vi "NF LI56xx sub get sig.vi"(7 "Type":string, 8 "error in":errorcluster caption="error in (no error)" {"code" format="%.0x"}, 10 "signal cluster":T1, 11 "VISA resource name":refnum<visa-resource-name>) -> (0 "error out":errorcluster {"code" format="%.0x"}, 2 "output":T1, 3 "VISA resource name copy":refnum<visa-resource-name>)   [LabVIEW 2019]
doc: "get input signal related parameters"
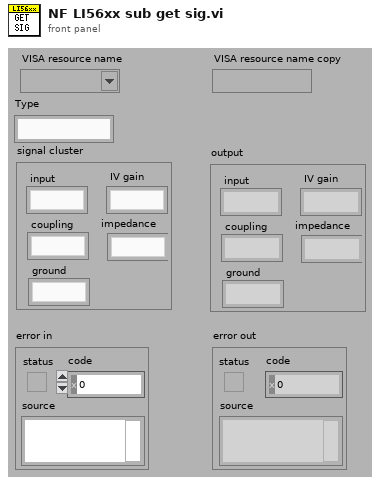
[diagram p1: front panel]
types:
  T1 = cluster{"input":string, "coupling":string, "ground":string, "IV gain":string, "impedance":string}
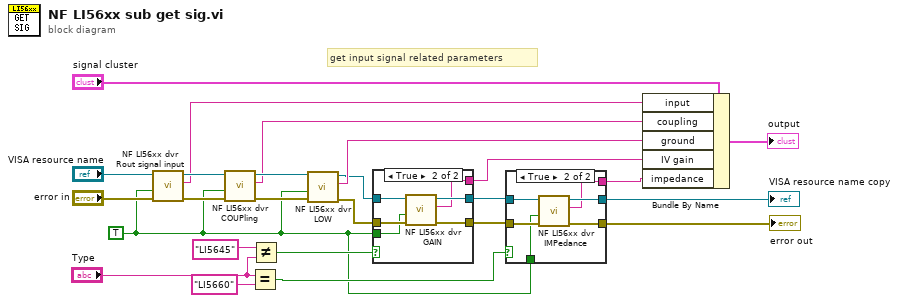
[diagram p0: block diagram]
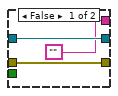
[diagram p2: hidden frame]
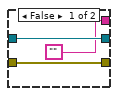
[diagram p3: hidden frame]
diagram:
  w1 = TRUE ("Read(F)")
  # "get input signal related parameters"
  n1 = call "NF LI56xx dvr Rout signal input.vi"("error in"="error in", "Read(F)"=w1, "VISA resource name"="VISA resource name") -> ("error out"=w23:errorcluster, "query signal input"=w19:string, "VISA resource name copy"=w25:refnum<visa-resource-name>)  [unwired: 6 in]
  n2 = call "NF LI56xx dvr COUPling.vi"("error in"=w23, "Read(F)"=w1, "VISA resource name"=w25) -> ("error out"=w22:errorcluster, "query coupling"=w18:string, "VISA resource name copy"=w24:refnum<visa-resource-name>)  [unwired: 6 in]
  n3 = Equal?(x="Type", y="LI5660") -> (x = y?=w8:bool)
  n4 = Not Equal?(x="LI5645" ("y"), y="Type") -> (x != y?=w7:bool)
  n5 = call "NF LI56xx dvr LOW.vi"("error in"=w22, "Read(F)"=w1, "VISA resource name"=w24) -> ("error out"=w4:errorcluster, "query grounding"=w17:string, "VISA resource name copy"=w5:refnum<visa-resource-name>)  [unwired: 6 in]
  n6 = case shown="True" w7 {
    tunnel: w5 -> [w28 w34]
    tunnel: w4 -> [w27 w33]
    tunnel: [w27 w32] -> w2
    tunnel: [w28 w31] -> w3
    tunnel: ["" w30] -> w6
    tunnel: w1 -> [_ w29]
    frame False {
    }
    frame True {
      n7 = call "NF LI56xx dvr GAIN.vi"("error in"=w33, "Read(F)"=w29, "VISA resource name"=w34) -> ("error out"=w32:errorcluster, "query IV gain"=w30:string, "VISA resource name copy"=w31:refnum<visa-resource-name>)  [unwired: 6 in]
    }
  }
  n8 = case shown="True" w8 {
    tunnel: w3 -> [w37 w43]
    tunnel: w2 -> [w36 w42]
    tunnel: [w36 w41] -> w13
    tunnel: [w37 w40] -> w12
    tunnel: ["" w39] -> w11
    tunnel: w1 -> [_ w38]
    frame False {
    }
    frame True {
      n9 = call "NF LI56xx dvr IMPedance.vi"("error in"=w42, "Read(F)"=w38, "VISA resource name"=w43) -> ("error out"=w41:errorcluster, "query input impedance"=w39:string, "VISA resource name copy"=w40:refnum<visa-resource-name>)  [unwired: 6 in]
    }
  }
  "error out" <- w13
  "VISA resource name copy" <- w12
  n10 = Bundle By Name(cluster="signal cluster", "input"=w19, "coupling"=w18, "ground"=w17, "IV gain"=w6, "impedance"=w11) -> (→"output":T1)
